vi "SetCurrentSource.vi"() -> ()   [LabVIEW 2018]
uses:
  <vilib>/Instr/_visa.llb/VISA Configure Serial Port (Instr).vi
  <vilib>/Utility/file.llb/Write Delimited Spreadsheet (DBL).vi
panel:
  in  "Current Scaling Factor 4":dbl=1.0 format="%#_13g"
  in  "Current Scaling Factor 3":dbl=1.0 format="%#_13g"
  in  "Current Scaling Factor 2":dbl=1.0 format="%#_13g"
  in  "Current Offset Amount 4":dbl format="%#_13g"
  in  "Current Offset Amount 3":dbl format="%#_13g"
  in  "Current Offset Amount 2":dbl format="%#_13g"
  in  "Gain Sel":bool=TRUE
  in  "Current Offset Amount":dbl format="%#_13g"
  out "OPT_PWR_MV":dbl format="%#_13g"
  in  "30 dB Power Conversion Factor":dbl=0.0531
  in  "Optical  Scaling Factor":dbl=4.0
  in  "20 dB Power Conversion Factor":dbl=0.1692
  out "Settings read string":string
  out "Settings reply":string
  out "Settings string":string
  out "ADC read string":string
  in  "Voltage stop (mV)":dbl=20000.0 format="%#_13g"
  out "Saved location and filename":path
  in  "Filename and location":path
  in  "Current Scaling Factor":dbl=1.0 format="%#_13g"
  in  "Loop length (ms)":i32=1000
  in  "Voltage step (mV)":dbl=50.0 format="%#_13g"
  out "Voltage (mV)":dbl
  out "Pulse Width":dbl
  out "Frequency":dbl
  out "ACD 2":dbl
  out "ADC 3":dbl
  out "ADC 4":dbl
  out "ADC 1":dbl
  out "RAW 3":dbl
  out "RAW 2":dbl
  out "RAW 4":dbl
  out "RAW 1":dbl
  out "Running?":bool
  in  "ON/OFF":bool
  in  "Voltage start (mV)":dbl=800.0
  in  "Pulse Width (ns)":dbl=3000.0
  in  "Frequency (Hz)":dbl=1000.0
  out "error out":errorcluster
  in  "VISA resource name":refnum<visa-resource-name>
  in  "error in (no error)":errorcluster
  out "VISA resource name out":refnum<visa-resource-name>
  # "CONFIG"
  # "DEVICE DATA"
  # "OUTPUT SETTINGS"
  # "DEBUG:"
  # "mA"
  # "mV"
  # "SWEEP SETTINGS"
  # "OUTPUT ENABLE"
  # "OPTICAL SENSOR CONFIG"
  # "CURRENT CALIBRATION"
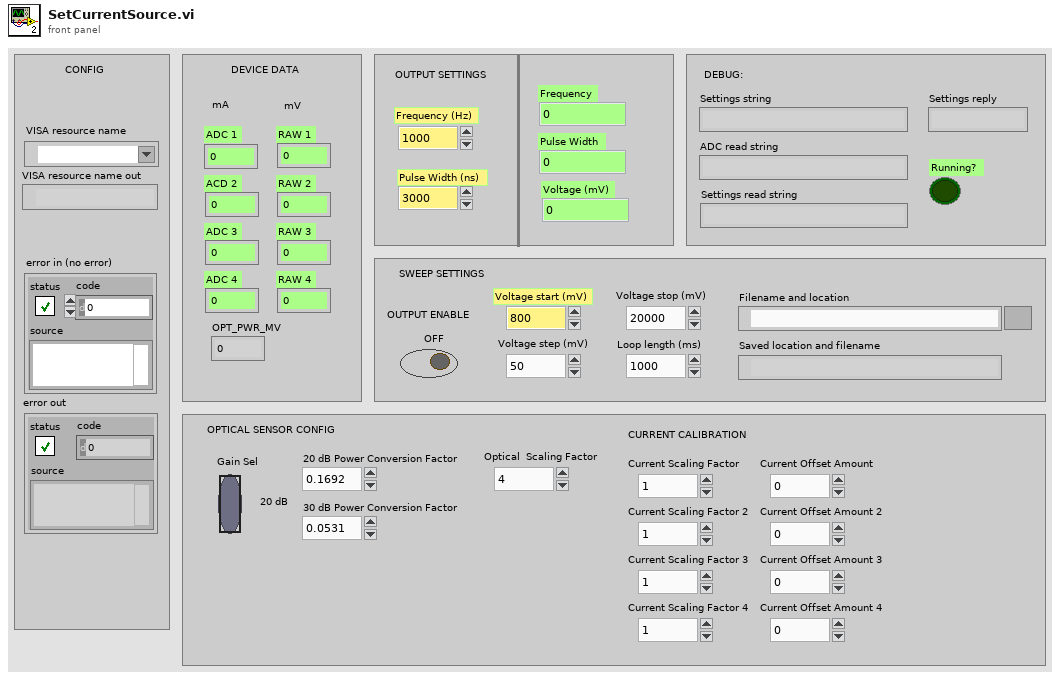
[diagram p1: front panel]
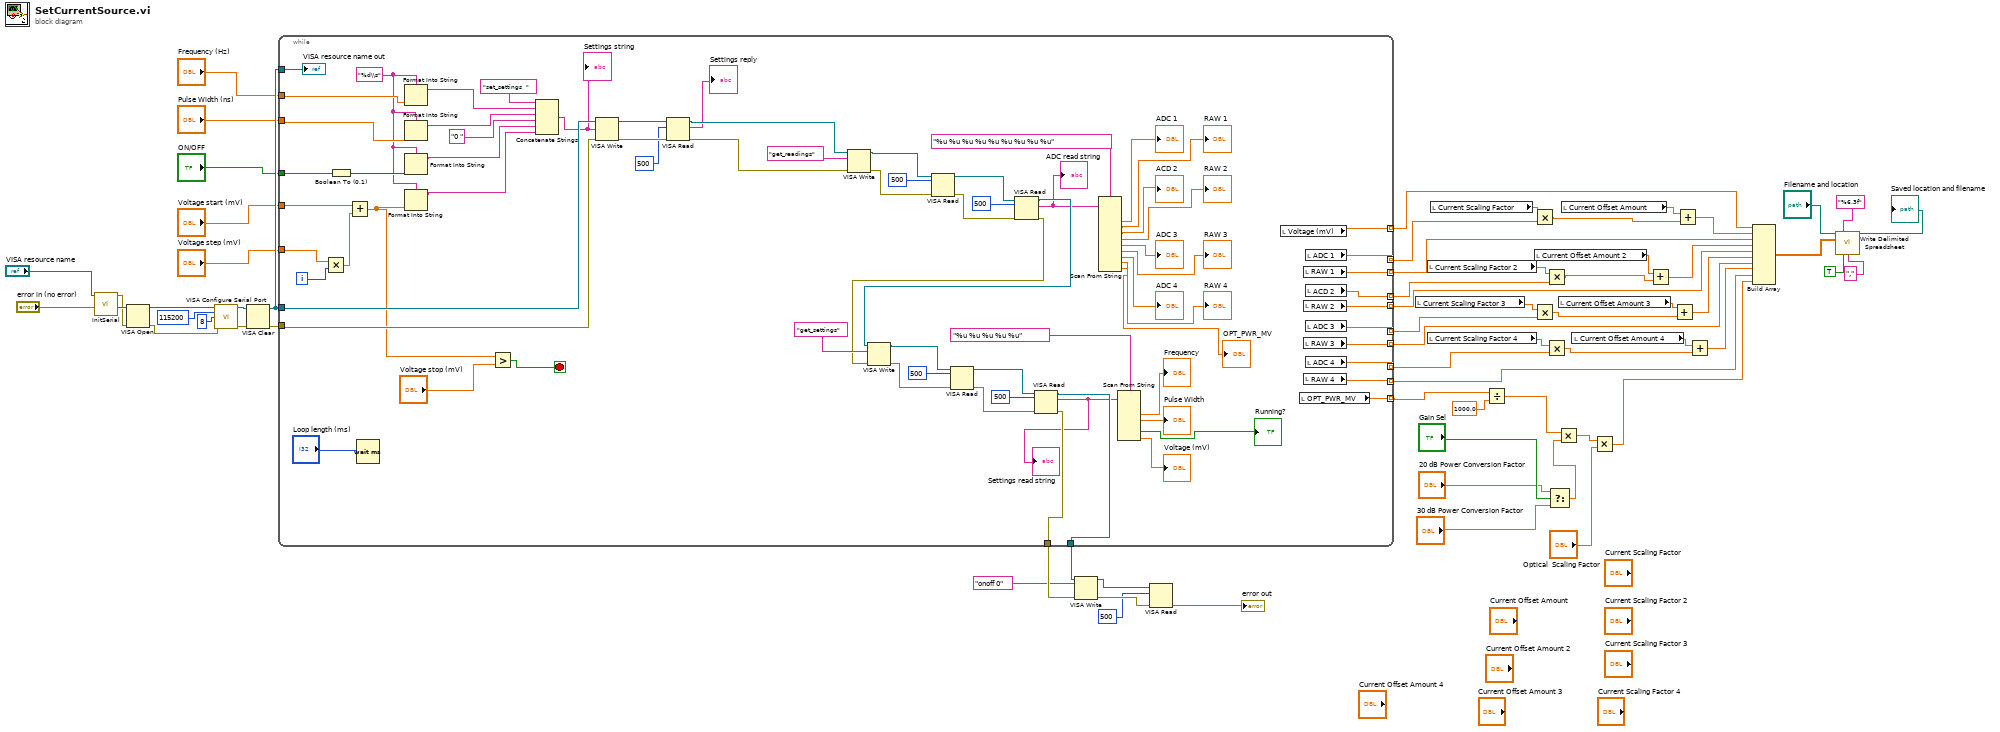
[diagram p0: block diagram]
diagram:
  n1 = call "InitSerial.vi"("error in (no error)"="error in (no error)", "VISA resource name"="VISA resource name") -> ("VISA resource name out"=w63:refnum<visa-resource-name>, "error out"=w55:errorcluster)  [unwired: 8 in]
  n2 = VISA Open(error in (no error)=w55, VISA resource name=w63) -> (VISA resource name=w62:refnum<visa-resource-name>, error out=w54:errorcluster)  [unwired: 3 in]
  n3 = call-poly "VISA Configure Serial Port"("VISA resource name"=w62, "baud rate (9600)"=115200, "data bits (8)"=8, "error in (no error)"=w54) -> ("VISA resource name out"=w58:refnum<visa-resource-name>, "error out"=w59:errorcluster)  [unwired: 10 in]
  n4 = VISA Clear(VISA resource name=w58, error in (no error)=w59) -> (VISA resource name out=w57:refnum<visa-resource-name>, error out=w56:errorcluster)
  n5 = while {
    tunnel: w56 -> [w83]
    tunnel: w57 -> [w139]
    tunnel: w57 -> [w84]
    tunnel: "Voltage start (mV)" -> [w111]
    tunnel: "Pulse Width (ns)" -> [w89]
    tunnel: "Frequency (Hz)" -> [w91]
    tunnel: "Voltage step (mV)" -> [w110]
    tunnel: "ON/OFF" -> [w105]
    tunnel: [w104] -> w48
    tunnel: [w103] -> w47
    tunnel: [w95] -> w17 mode=indexing
    tunnel: [w100] -> w41 mode=indexing
    tunnel: [w92] -> w19 mode=indexing
    tunnel: [w96] -> w37 mode=indexing
    tunnel: [w93] -> w13 mode=indexing
    tunnel: [w97] -> w38 mode=indexing
    tunnel: [w94] -> w15 mode=indexing
    tunnel: [w98] -> w39 mode=indexing
    tunnel: [w99] -> w40 mode=indexing
    tunnel: [w66] -> w22 mode=indexing
    i -> [w107]
    stop <- w75 stop-if-true
    w88 = "%d\\s"
    n6 = Multiply(x=w110, y=w107) -> (x*y=w106:dbl)
    n7 = Boolean To (0,1)(Boolean=w105) -> (0, 1=w90:i16)
    n8 = Add(x=w111, y=w106) -> (x+y=w76:dbl)
    n9 = Wait (ms)(milliseconds to wait="Loop length (ms)") -> ()  [unwired: 1 out]
    n10 = Format Into String(format string=w88, w91) -> (resulting string=w86:string)  [unwired: 2 in, 1 out]
    n11 = Format Into String(format string=w88, w89) -> (resulting string=w85:string)  [unwired: 2 in, 1 out]
    n12 = Format Into String(format string=w88, w90) -> (resulting string=w73:string)  [unwired: 2 in, 1 out]
    n13 = Format Into String(format string=w88, w76) -> (resulting string=w74:string)  [unwired: 2 in, 1 out]
    n14 = Greater?(x=w76, y="Voltage stop (mV)") -> (0:w75:bool)
    n15 = Concatenate Strings("set_settings  ", w86, w85, "0 ", w73, w74) -> (w70:string)
    "Settings string" <- w70
    n16 = VISA Write(VISA resource name=w84, write buffer=w70, error in (no error)=w83) -> (VISA resource name out=w81:refnum<visa-resource-name>, error out=w82:errorcluster)  [unwired: 1 out]
    n17 = VISA Read(VISA resource name=w81, byte count=500, error in (no error)=w82) -> (VISA resource name out=w79:refnum<visa-resource-name>, read buffer=→"Settings reply":string, error out=w78:errorcluster)  [unwired: 1 out]
    n18 = VISA Write(VISA resource name=w79, write buffer="get_readings", error in (no error)=w78) -> (VISA resource name out=w134:refnum<visa-resource-name>, error out=w136:errorcluster)  [unwired: 1 out]
    n19 = VISA Read(VISA resource name=w134, byte count=500, error in (no error)=w136) -> (VISA resource name out=w131:refnum<visa-resource-name>, error out=w133:errorcluster)  [unwired: 2 out]
    n20 = VISA Read(VISA resource name=w131, byte count=500, error in (no error)=w133) -> (VISA resource name out=w114:refnum<visa-resource-name>, read buffer=w71:string, error out=w113:errorcluster)  [unwired: 1 out]
    "ADC read string" <- w71
    n21 = VISA Write(VISA resource name=w114, write buffer="get_settings", error in (no error)=w113) -> (VISA resource name out=w122:refnum<visa-resource-name>, error out=w121:errorcluster)  [unwired: 1 out]
    n22 = VISA Read(VISA resource name=w122, byte count=500, error in (no error)=w121) -> (VISA resource name out=w124:refnum<visa-resource-name>, error out=w123:errorcluster)  [unwired: 2 out]
    n23 = VISA Read(VISA resource name=w124, byte count=500, error in (no error)=w123) -> (VISA resource name out=w103:refnum<visa-resource-name>, read buffer=w68:string, error out=w104:errorcluster)  [unwired: 1 out]
    "Settings read string" <- w68
    n24 = Scan From String(format string="%u %u %u %u %u %u %u %u %u", input string=w71) -> (output 1=→"ADC 1":dbl, output 2=→"RAW 1":dbl, output 3=→"ACD 2":dbl, output 4=→"RAW 2":dbl, output 5=→"ADC 3":dbl, output 6=→"RAW 3":dbl, output 7=→"ADC 4":dbl, output 8=→"RAW 4":dbl, output 9=→"OPT_PWR_MV":dbl)  [unwired: 11 in, 3 out]
    n25 = Scan From String(format string="%u %u %u %u %u", input string=w68) -> (output 1=→"Frequency":dbl, output 2=→"Pulse Width":dbl, output 4=→"Running?":bool, output 5=→"Voltage (mV)":dbl)  [unwired: 8 in, 3 out]
    n26 = local read "Voltage (mV)"() -> (w100:dbl)
    n27 = local read "OPT_PWR_MV"() -> (w66:dbl)
    n28 = local read "RAW 1"() -> (w96:dbl)
    n29 = local read "RAW 2"() -> (w97:dbl)
    n30 = local read "RAW 3"() -> (w98:dbl)
    n31 = local read "RAW 4"() -> (w99:dbl)
    n32 = local read "ADC 1"() -> (w92:dbl)
    n33 = local read "ACD 2"() -> (w93:dbl)
    n34 = local read "ADC 3"() -> (w94:dbl)
    n35 = local read "ADC 4"() -> (w95:dbl)
    "VISA resource name out" <- w139
  }
  n36 = VISA Write(VISA resource name=w47, write buffer="onoff 0", error in (no error)=w48) -> (VISA resource name out=w45:refnum<visa-resource-name>, error out=w44:errorcluster)  [unwired: 1 out]
  n37 = VISA Read(VISA resource name=w45, byte count=500, error in (no error)=w44) -> (error out=→"error out":errorcluster)  [unwired: 3 out]
  n38 = local read "Current Scaling Factor 3"() -> (w16:dbl)
  n39 = local read "Current Scaling Factor 2"() -> (w14:dbl)
  n40 = local read "Current Scaling Factor 4"() -> (w18:dbl)
  n41 = local read "Current Scaling Factor"() -> (w20:dbl)
  n42 = Divide(x=w22, y=1000.0) -> (x/y=w21:dbl[])
  n43 = Multiply(x=w20, y=w19) -> (x*y=w10:dbl[])
  n44 = Multiply(x=w16, y=w15) -> (x*y=w5:dbl[])
  n45 = local read "Current Offset Amount 2"() -> (w9:dbl)
  n46 = Multiply(x=w14, y=w13) -> (x*y=w8:dbl[])
  n47 = Multiply(x=w18, y=w17) -> (x*y=w2:dbl[])
  n48 = Select(t="20 dB Power Conversion Factor", s="Gain Sel", f="30 dB Power Conversion Factor") -> (s? t:f=w27:dbl)
  n49 = Multiply(x=w21, y=w27) -> (x*y=w26:dbl[])
  n50 = local read "Current Offset Amount 3"() -> (w6:dbl)
  n51 = local read "Current Offset Amount"() -> (w12:dbl)
  n52 = local read "Current Offset Amount 4"() -> (w3:dbl)
  n53 = Multiply(x=w26, y="Optical  Scaling Factor") -> (x*y=w24:dbl[])
  n54 = Add(x=w9, y=w8) -> (x+y=w7:dbl[])
  n55 = Add(x=w6, y=w5) -> (x+y=w4:dbl[])
  n56 = Add(x=w12, y=w10) -> (x+y=w11:dbl[])
  n57 = Add(x=w3, y=w2) -> (x+y=w1:dbl[])
  n58 = Build Array(w41, w11, w37, w7, w38, w4, w39, w1, w40, w24) -> (w33:dbl[][])
  n59 = call-poly <vilib>:"Write Delimited Spreadsheet.vi"("file path (dialog if empty)"="Filename and location", "format (%.3f)"="%6.3f", "2D data"=w33, "transpose? (no:F)"=TRUE, "delimiter (\\t)"=",") -> ("new file path (Not A Path if cancelled)"=→"Saved location and filename":path)  [unwired: 9 in, 1 out]
